vi "WallFollow.vi"(3 "SupressIn":dbl, 7 "Inhibit":bool, 8 "HowAmI? Clean":cluster{"T":dbl, "Battery":dbl, "Temp":dbl}, 9 "WhatAroundMe? Clean":cluster{"T":dbl, "Range":dbl, "Bearing":dbl}[](array[cluster]), 10 "WhereAmI? Clean":T2, 11 "Velocity":dbl) -> (0 "SupressOut":dbl, 2 "ActCommand":dbl[](array[numeric]), 4 "InhibitOut":bool)   [LabVIEW 2012]
doc: "This subVI executes a wall folowing Midbrain behaviors. Its inputs are the outputs of the three SENSE processes, the overall velocity requested of the robot, a suppression value from another co-brahvior and an inhibit signal to turn the behavior off. The outputs are a 90 element steering array, a suppression value to diminish the output of co-behaviors and an inhibit output to shut off otehr behaviors.\n\nIt is designed to work with a 90 element behavior arbiter."
uses:
  <vilib>/addons/control/pid/pid.llb/PID (DBL).vi
  <vilib>/addons/control/pid/NI_PID_pid.lvlib
panel:
  out "Waveform Chart":dbl(graph)
  out "steer":dbl format="%.2f"
  out "Range":dbl
  in  "PID gains":T1={"proportional gain (Kc)"=20.0, "integral time (Ti, min)"=0.008, "derivative time (Td, min)"=0.001} {"derivative time (Td, min)" format="%.3f"; "integral time (Ti, min)" format="%.3f"; "proportional gain (Kc)" format="%.3f"}
  # "This VI contains a wall following behavior at the Midbrain level"
  # "0.5"
  # "0"
  # "35"
  # "0"
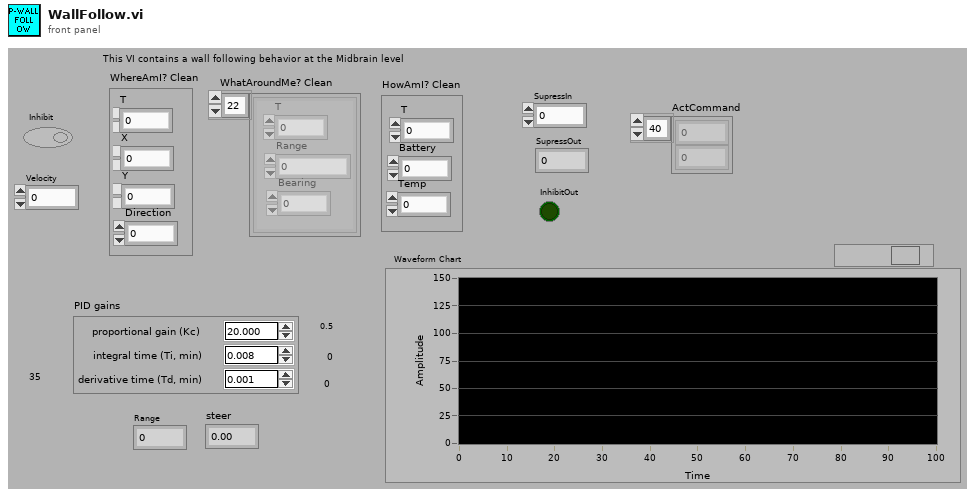
[diagram p1: front panel]
types:
  T1 = cluster{"proportional gain (Kc)":dbl, "integral time (Ti, min)":dbl, "derivative time (Td, min)":dbl}
  T2 = cluster{"T":dbl, "X":dbl, "Y":dbl, "Direction":dbl}
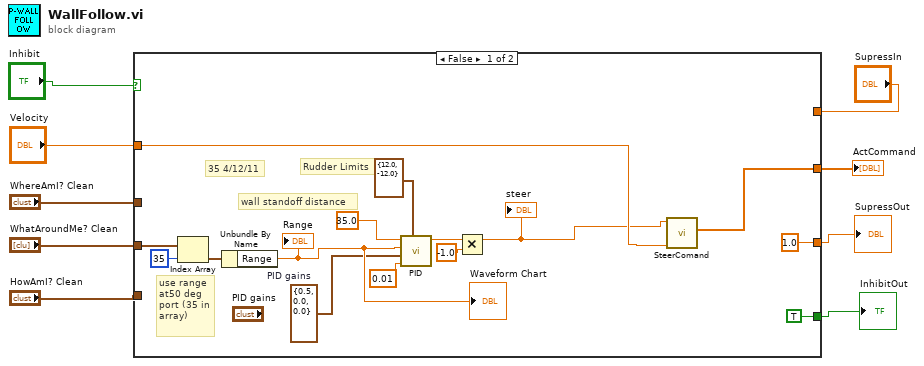
[diagram p0: block diagram]
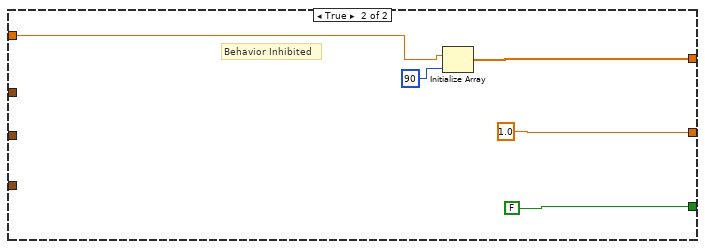
[diagram p2: hidden frame]
diagram:
  n1 = case shown="False" "Inhibit" {
    tunnel: "Velocity" -> [w20 w25]
    tunnel: "WhatAroundMe? Clean" -> [w22 _]
    tunnel: "WhereAmI? Clean" -> [_ _]
    tunnel: "HowAmI? Clean" -> [_ _]
    tunnel: "SupressIn" -> [_ _]
    tunnel: [w19 w27] -> w2
    tunnel: [1.0 ("SupressOut") 1.0 ("SupressOut")] -> w3
    tunnel: [TRUE ("InhibitOut") FALSE ("InhibitOut")] -> w1
    frame False {
      w10 = T1 {"proportional gain (Kc)"=0.5, "integral time (Ti, min)"=0.0, "derivative time (Td, min)"=0.0}  # PID gains
      # "35 4/12/11"
      # "Rudder Limits"
      # "wall standoff distance"
      # "use range \nat50 deg\nport (35 in\narray)"
      n2 = Index Array "Index Array"(array=w22, index=35) -> (element=w21:cluster{"T":dbl, "Range":dbl, "Bearing":dbl})
      n3 = Unbundle By Name(w21) -> ("Range"=w15:dbl)
      "Range" <- w15
      "Waveform Chart" <- w15
      n4 = call-poly <vilib>:"PID.vi"("output range"=cluster{"output high":dbl, "output low":dbl} {"output high"=12.0, "output low"=-12.0}, "dt (s)"=0.01, "PID gains"=w10, "process variable"=w15, "setpoint"=35.0) -> ("output"=w17:dbl)  [unwired: 5 in, 1 out]
      n5 = Multiply(x=w17, y=-1.0) -> (x*y=w14:dbl)
      "steer" <- w14
      n6 = call "SteerComand.vi"("Speed"=w20, "SteeringAngle"=w14) -> ("ManualActCommand"=w19:dbl[])  [unwired: 9 in]
    }
    frame True {
      # "Behavior Inhibited"
      n7 = Initialize Array "Initialize Array"(w25, 90 ("dimension size")) -> (w27:dbl[])
    }
  }
  "ActCommand" <- w2
  "SupressOut" <- w3
  "InhibitOut" <- w1
